vi "Globals.vi"() -> ()   [LabVIEW 2017, in "nifxpmath_Add.xnode"]
uses:
  <vilib>/rvi/FXPMathLib/FxpAdd/XNode/nifxpmath_Add.xnode
panel:
  out "SMALL ICON w/ 4WIRE":picture
  in  "TERM X+Y NAME":string="x+y"
  in  "TERM Y NAME":string="y"
  in  "TERM X NAME":string="x"
  in  "TERM OVFL ID":string="TERM_OVFL"
  in  "TERM X+Y ID":string="TERM_XY"
  in  "TERM Y ID":string="TERM_Y"
  in  "TERM X ID":string="TERM_X"
  out "SMALL ICON":picture
  out "NORMAL BANNER":picture
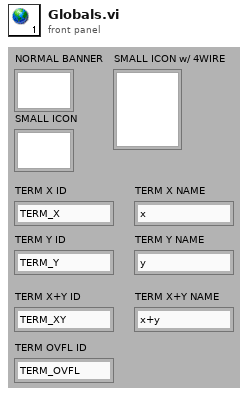
[diagram p1: front panel]
diagram:
